vi "Write Maximum Channel Duration.vi"(8 "error in (no error)":errorcluster, 10 "maximum channel duration (s)":dbl, 11 "Waveforms (N Ch) in":refnum<class "Waveforms (N Ch).lvclass">) -> (0 "error out":errorcluster, 3 "Waveforms (N Ch) out":refnum<class "Waveforms (N Ch).lvclass">)   [LabVIEW 2017, in "Waveforms (N Ch).lvclass"]
uses:
  <vilib>/addons/_NISVFA/_Shared subVIs/Data Objects/Waveforms (DBL)/Waveforms (N Ch).lvclass
  C:/Program Files (x86)/National Instruments/LabVIEW 2017/vi.lib/addons/_NISVFA/_Shared subVIs/Data Objects/Data/Data.lvclass
  <vilib>/addons/_NISVFA/_Shared subVIs/Data Objects/Data/Data.lvclass/Data.ctl
  <vilib>/addons/_NISVFA/_Shared subVIs/Data Objects/Data/Data.lvclass
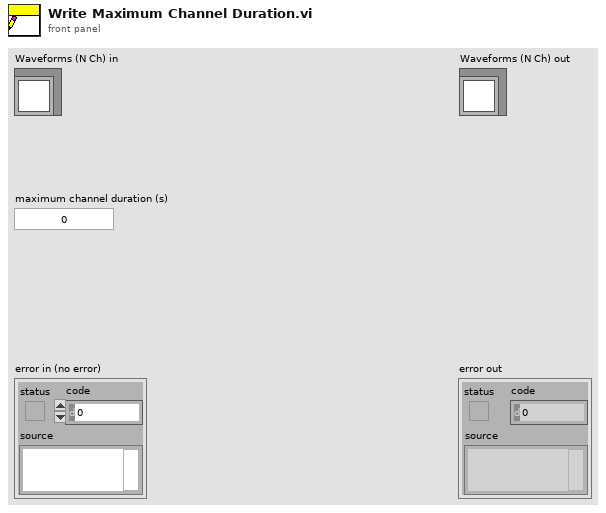
[diagram p1: front panel]
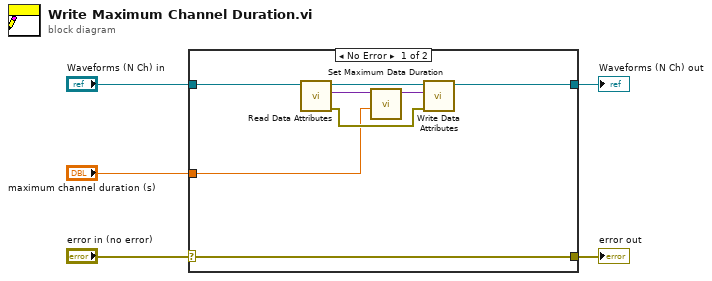
[diagram p0: block diagram]
diagram:
  n1 = case shown="No Error" "error in (no error)" {
    selector: "error in (no error)" -> [w13 w14]
    tunnel: [w13 w14] -> w4
    tunnel: [w10 w15] -> w2
    tunnel: "Waveforms (N Ch) in" -> [w12 w15]
    tunnel: "maximum channel duration (s)" -> [w6 _]
    frame No Error {
      n2 = call <vilib>:"Read Data Attributes.vi"("Data in"=w12) -> ("error out"=w7:errorcluster, "data attributes"=w9:variant, "Data out"=w11:refnum<class "Waveforms (N Ch).lvclass">)  [unwired: 8 in]
      n3 = call <vilib>:"Set Maximum Data Duration.vi"("maximum data duration"=w6, "variant in"=w9) -> ("variant out"=w8:variant)  [unwired: 9 in]
      n4 = call <vilib>:"Write Data Attributes.vi"("error in (no error)"=w7, "data attributes"=w8, "Data in"=w11) -> ("Data out"=w10:refnum<class "Waveforms (N Ch).lvclass">)  [unwired: 7 in, 1 out]
    }
    frame Error {
    }
  }
  "error out" <- w4
  "Waveforms (N Ch) out" <- w2
